vi "Arithmetic.vi"() -> ()   [LabVIEW 2014]
panel:
  out "Result10":dbl format="%_6g"
  in  "h":i32
  out "Result9":dbl
  out "Result8":dbl
  in  "g":dbl
  in  "f":dbl
  out "Result7":dbl
  out "Result6":dbl
  in  "e":dbl
  in  "d":dbl
  out "Result5":dbl
  out "Result4":dbl
  out "Result3":dbl
  out "Result2":dbl
  out "Result1":dbl
  in  "c":dbl
  in  "b":dbl
  in  "a":dbl
  # "a+b="
  # "a-b="
  # "a*b="
  # "a/b="
  # "(a+b)*c="
  # "Remainder(d/e)"
  # "Quotient(d/e)"
  # "sqrt(f)"
  # "g^2"
  # "dbl(h)"
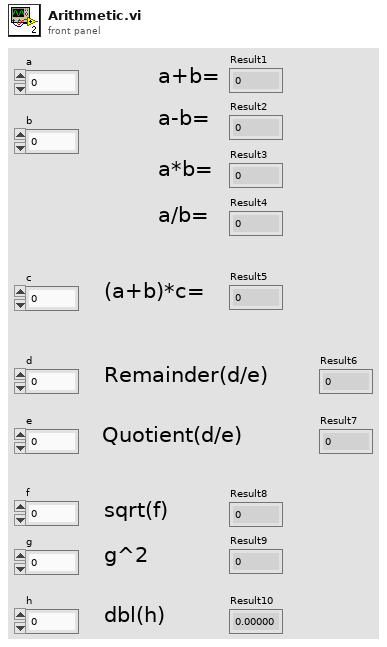
[diagram p1: front panel]
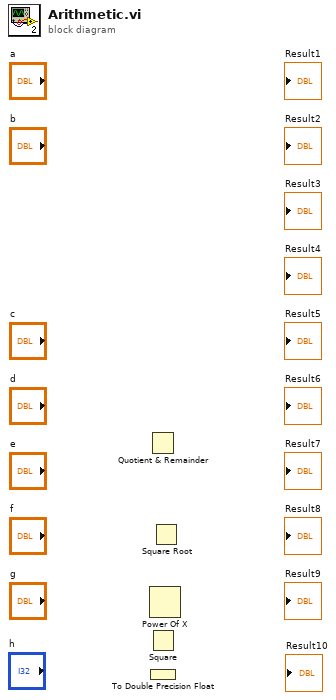
[diagram p0: block diagram]
diagram:
  n1 = Quotient & Remainder() -> ()  [unwired: 2 in, 2 out]
  n2 = Square() -> ()  [unwired: 1 in, 1 out]
  n3 = To Double Precision Float() -> ()  [unwired: 1 in, 1 out]
  n4 = Power Of X() -> ()  [unwired: 2 in, 1 out]
  n5 = Square Root() -> ()  [unwired: 1 in, 1 out]
